vi "ImpulseData - Get Saccade Trace.vi"(0 "Saccade in":T1, 1 "Pre Surround idx (0)":i32, 2 "Post Surround idx (0)":i32, 3 "error in (no error)":errorcluster, 4 "Impulse Data":refnum<data-value>) -> (7 "Saccade out":T1, 8 "Response Data":dbl[](array[numeric]), 9 "Stimulus Data":dbl[](array[numeric]), 10 "error out":errorcluster)   [LabVIEW 2016]
uses:
  Type Definitions/Saccade Analyser Saccade Data.ctl
  Type Definitions/Saccade Analyser Impulse Data.ctl
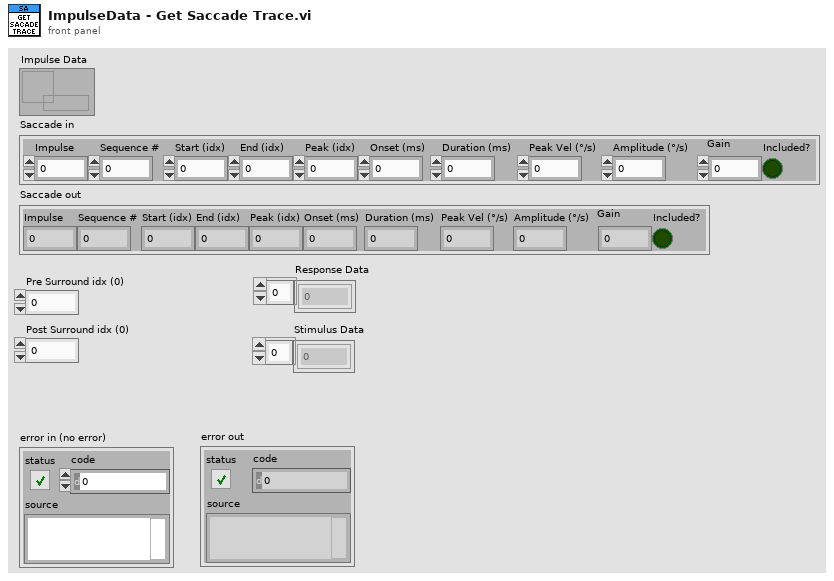
[diagram p1: front panel]
types:
  T1 = typedef "Saccade Analyser Saccade Data.ctl" = cluster{"Impulse":i32, "Sequence #":dbl, "Start (idx)":dbl, "End (idx)":dbl, "Peak (idx)":dbl, "Onset (ms)":dbl, "Duration (ms)":dbl, "Peak Vel (°/s)":dbl, "Amplitude (°/s)":dbl, "Gain":dbl, "Included?":bool}
  T2 = typedef "Saccade Analyser Impulse Data.ctl" = cluster{"Stimulus Data":dbl[], "Response Data":dbl[], "Peak (idx)":i32, "Onset (idx)":i32}
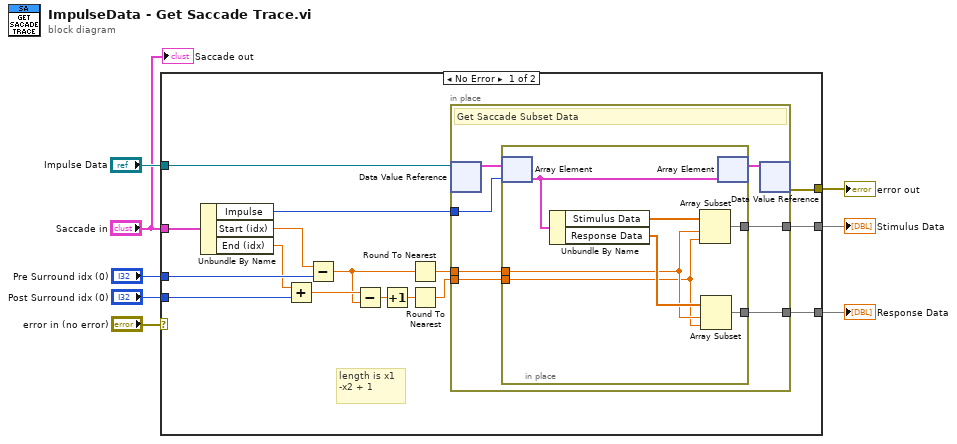
[diagram p0: block diagram]
diagram:
  n1 = case shown="No Error" "error in (no error)" {
    selector: "error in (no error)" -> [_ w39]
    tunnel: "Impulse Data" -> [w24 _]
    tunnel: "Saccade in" -> [w23 _]
    tunnel: "Pre Surround idx (0)" -> [w20 _]
    tunnel: "Post Surround idx (0)" -> [w18 _]
    tunnel: [w14 _] -> w3
    tunnel: [w13 _] -> w2
    tunnel: [w12 w39] -> w1
    frame No Error {
      # "length is x1 -x2 + 1"
      n2 = Unbundle By Name(w23) -> ("Impulse"=w22:i32, "Start (idx)"=w21:dbl, "End (idx)"=w19:dbl)
      n3 = Add(x=w19, y=w18) -> (x+y=w17:dbl)
      n4 = Subtract(x=w21, y=w20) -> (x-y=w16:dbl)
      n5 = Subtract(x=w17, y=w16) -> (x-y=w15:dbl)
      n6 = Increment(x=w15) -> (x+1=w9:dbl)
      n7 = Round To Nearest(number=w16) -> (nearest integer value=w11:dbl)
      n8 = Round To Nearest(number=w9) -> (nearest integer value=w10:dbl)
      n9 = in-place {
        in-place-border: w22 -> [w29]
        in-place-border: w11 -> [w28]
        in-place-border: w10 -> [w27]
        in-place-border: [w26] -> w14
        in-place-border: [w25] -> w13
        # "Get Saccade Subset Data"
        n10 = in-place-dvr #1(w24) -> (w31:T2[])  [unwired: 1 out]
        n11 = in-place {
          in-place-border: w28 -> [w34]
          in-place-border: w27 -> [w33]
          in-place-border: [w36] -> w26
          in-place-border: [w32] -> w25
          n12 = in-place-array #2(w31, w29) -> (w38:T2)
          n13 = Unbundle By Name(w38) -> ("Stimulus Data"=w37:dbl[], "Response Data"=w35:dbl[])
          n14 = Array Subset(array=w37, index=w34, length=w33) -> (w36:dbl[])
          n15 = Array Subset(array=w35, index=w34, length=w33) -> (w32:dbl[])
          n16 = in-place-array #2(w38) -> (w30:T2[])  [unwired: 1 out]
        }
        n17 = in-place-dvr #1(w30) -> (w12:errorcluster)  [unwired: 1 out]
      }
    }
    frame Error {
    }
  }
  "error out" <- w1
  "Response Data" <- w2
  "Stimulus Data" <- w3
  "Saccade out" <- "Saccade in"
